vi "ADQ214 Set Afe Switch.vi"(8 "error in (no error)":errorcluster, 9 "afemask":u32, 10 "adq214_num":i32, 11 "adq_cu_ptr":u32) -> (0 "error out":errorcluster, 2 "function return":i32, 3 "adq_cu_ptr out":u32)   [LabVIEW 2013]
doc: "extern \"C\" __declspec(dllimport) int ADQ214_SetAfeSwitch(void* adq_cu_ptr, int adq214_num, unsigned int afemask);"
uses:
  dlls/ADQAPI.dll
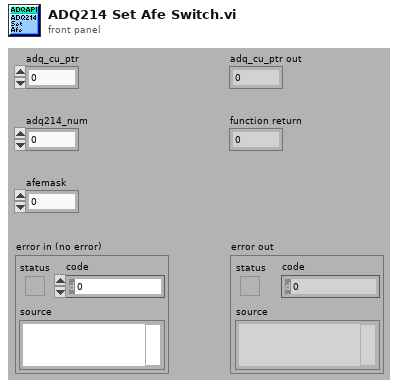
[diagram p1: front panel]
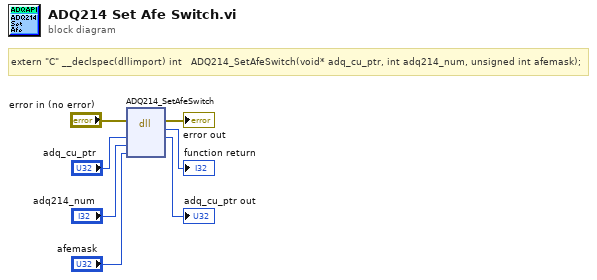
[diagram p0: block diagram]
diagram:
  # "extern \"C\" __declspec(dllimport) int\t\t\tADQ214_SetAfeSwitch(void* adq_cu_ptr, int adq214_num, unsigned int afemask);"
  n1 = dll-call lib="C:/Users/astafiev/Desktop/IlyaDrive/@photonCounting/LabView_Imperium/dlls/ADQAPI.*" fn="ADQ214_SetAfeSwitch"(error in="error in (no error)", "adq_cu_ptr"="adq_cu_ptr", "adq214_num"="adq214_num", "afemask"="afemask") -> (error out=→"error out":errorcluster, "return type"=→"function return":i32, "adq_cu_ptr"=→"adq_cu_ptr out":u32)  [unwired: 4 in, 1 out]
